vi "BB INV B Current Sense.vi"(8 "error in (no error)":errorcluster) -> (0 "Array":errorcluster[](array[cluster]), 3 "Current Readings":dbl[](array[numeric]))   [LabVIEW 2022 SP3]
uses:
  Serial Board Com/Board Select.ctl
  Serial Board Com/ADCSelector BB.ctl
panel:
  in  "Board Selector":T1
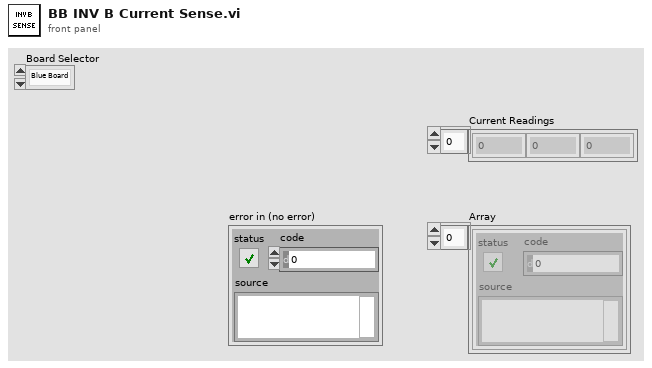
[diagram p1: front panel]
types:
  T1 = typedef "Board Select.ctl" = enum16{"Blue Board", "Green Board"}
  T2 = typedef "ADCSelector BB.ctl" = enum16{"INVA_ISENSE_U", "INVA_ISENSE_V", "INVA_ISENSE_W", "INVA_UDC", "INVA_TEMP", "HB_TEMP", "AUXB_TEMP", "VLINE_AB", "VLINE_BC", "VLINE_CA", "VSENSE_POS_24V", "VSENSE_POS_5V", "VSENSE_NEG_15V", "INVB_ISENSE_U", "INV_B_ISENSEV", "INVB_ISENSE_W", "INVB_UDC", "INVB_TEMP", "AUXA_TEMP", "AUXC_TEMP", "VOUT_AB", "VOUT_BC", "VOUT_CA", "VSENSE_POS_15V", "VSENSE_POS_3P3V", "TEST_POINT"}
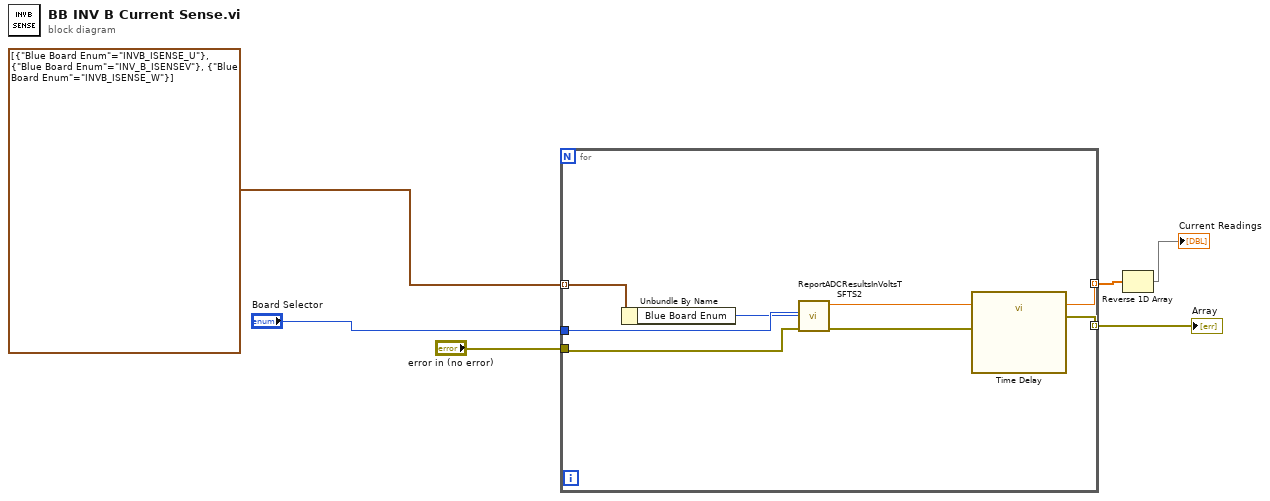
[diagram p0: block diagram]
diagram:
  n1 = for {
    tunnel: cluster{"Blue Board Enum":T2}[] [{"Blue Board Enum"=enum."INVB_ISENSE_U"}, {"Blue Board Enum"=enum."INV_B_ISENSEV"}, {"Blue Board Enum"=enum."INVB_ISENSE_W"}] -> [w11] mode=indexing
    tunnel: [w13] -> w6 mode=indexing
    tunnel: [w7] -> w5 mode=indexing
    tunnel: "error in (no error)" -> [w12]
    tunnel: "Board Selector" -> [w10]
    n2 = Unbundle By Name(w11) -> ("Blue Board Enum"=w9:T2)
    n3 = call "ReportADCResultsInVoltsTSFTS2.vi"("Blue Board Enum"=w9, "error in (no error)"=w12, "Board Selector"=w10) -> ("error out"=w8:errorcluster, "Result"=w13:dbl)  [unwired: 5 in, 2 out]
    n4 = call "Time Delay"("error in (no error)"=w8) -> ("error out"=w7:errorcluster)  [unwired: 10 in]
  }
  "Array" <- w5
  n5 = Reverse 1D Array(array=w6) -> (reversed array=→"Current Readings":dbl[])
